vi "Parse Path Object Items.vi"(9 "error in (no error)":errorcluster, 11 "Path with leading Object element":string) -> (1 "error out":errorcluster, 2 "<JSON>items names":string[](array[string]), 3 "Rest or Path":string, 4 "Is Array":bool)   [LabVIEW 2019, in "JSONtext.lvlib"]
uses:
  JSONtext.lvlib
  Parsing State.ctl
  Advance past Line Ending.vi
  support/quote and escape json string 2.vi
  JDP Science Common Utilities/JDP Utility.lvlib
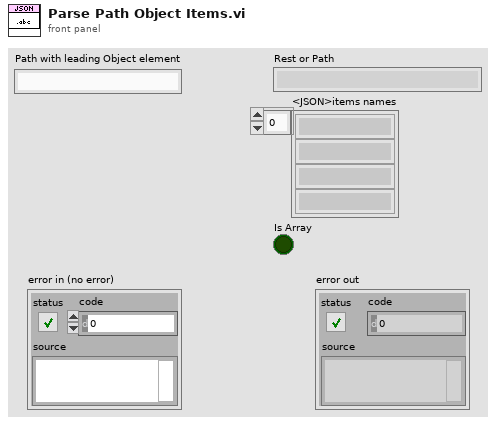
[diagram p1: front panel]
types:
  T1 = typedef "JSONtext.lvlib/Parsing State.ctl" = enum16{"Parser Error", "Object", "Array", "String", "Number/Other", "Leading Whitespace", "Object end", "Array end", "Value end"}
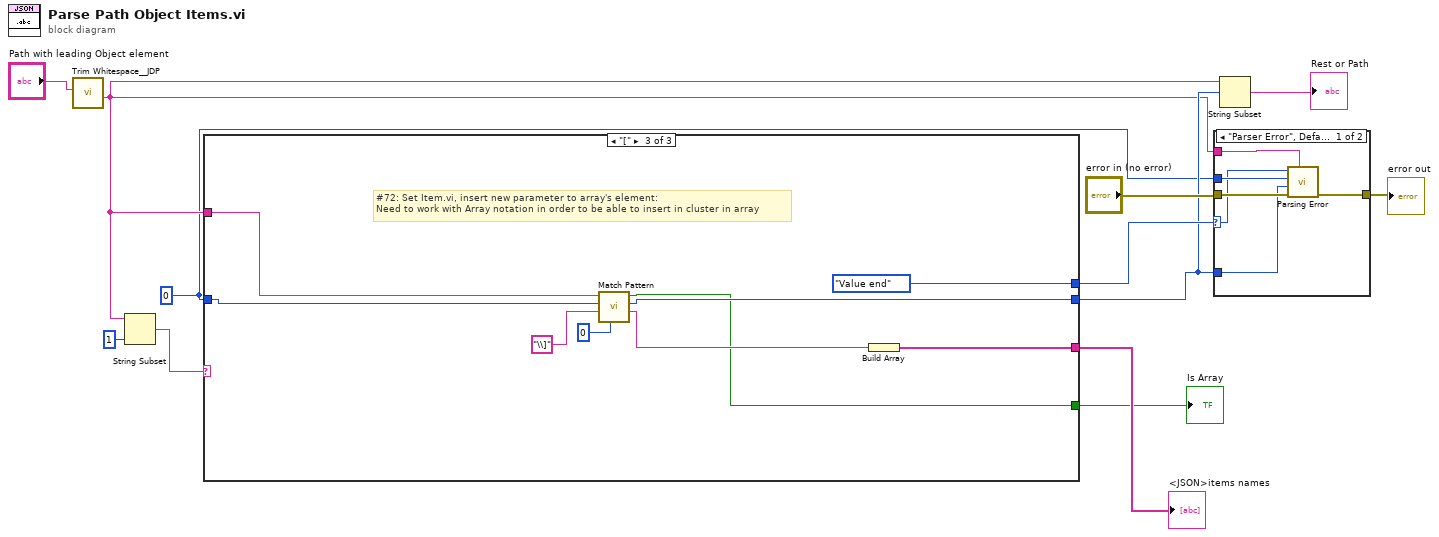
[diagram p0: block diagram]
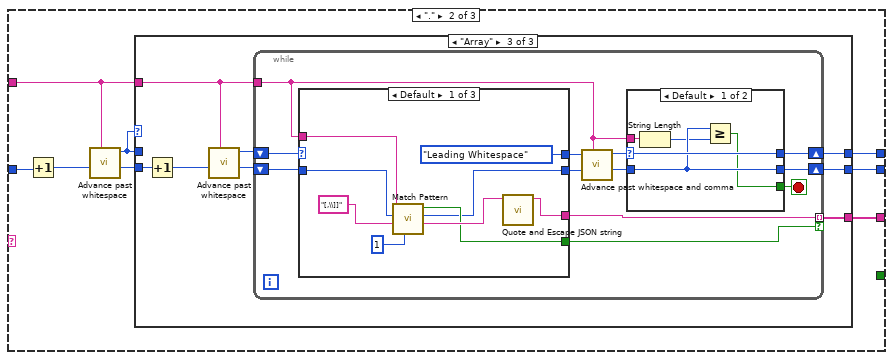
[diagram p4: hidden frame]
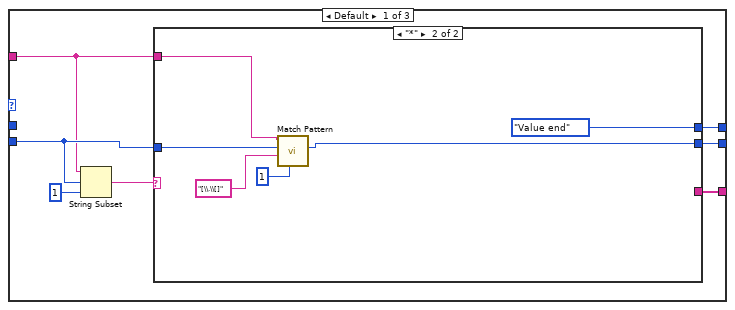
[diagram p5: hidden frame]
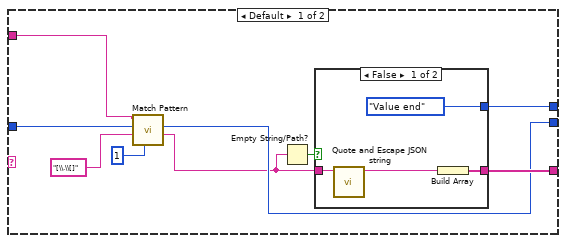
[diagram p6: hidden frame]
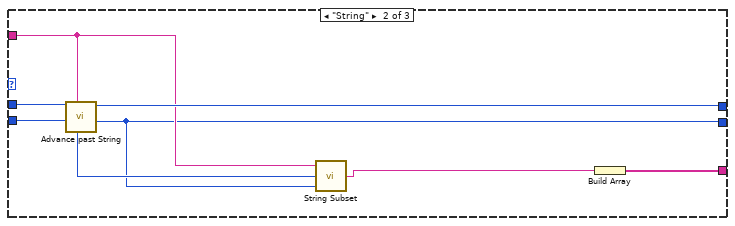
[diagram p8: hidden frame]
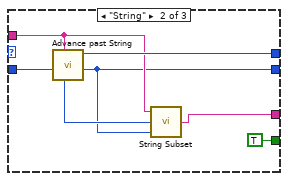
[diagram p9: hidden frame]
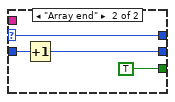
[diagram p11: hidden frame]
diagram:
  w3 = 0
  n1 = call "Trim Whitespace__JDP.vi"("String in"="Path with leading Object element") -> ("String out"=w5:string)  [unwired: 6 in]
  n2 = String Subset(string=w5, length (rest)=1 ("length (rest)")) -> (substring=w2:string)  [unwired: 1 in]
  n3 = case shown="\"[\"" w2 {
    tunnel: w3 -> [w13 w21 w111]
    tunnel: w5 -> [_ w19 w110]
    tunnel: [_ w18 w104] -> w9
    tunnel: [w13 w17 w109] -> w8
    tunnel: [_ w14 Parsing_State."Value end" ("Parser State")] -> w10
    tunnel: [_ _ w103] -> w1
    frame Default {
    }
    frame "." {
      n4 = Increment(x=w21) -> (x+1=w20:i32)
      n5 = call "Advance past whitespace.vi"("JSON"=w19, "Offset"=w20) -> ("Offset of first non-whitespace"=w16:i32, "Parser State"=w15:T1)  [unwired: 7 in, 1 out]
      n6 = case shown="\"Array\"" w15 {
        tunnel: w15 -> [_ w55 _]
        tunnel: w19 -> [w23 w52 w56]
        tunnel: w16 -> [w24 w54 w63]
        tunnel: [w28 w48 w62] -> w18
        tunnel: [w27 w50 w61] -> w17
        tunnel: [w26 w53 w60] -> w14
        frame Default {
          n7 = String Subset(string=w23, offset (0)=w24, length (rest)=1 ("length (rest)")) -> (substring=w22:string)
          n8 = case shown="\"*\"" w22 {
            tunnel: [w37 _] -> w28
            tunnel: [w35 w46] -> w27
            tunnel: [w34 Parsing_State."Value end" ("Parser State")] -> w26
            tunnel: w24 -> [w30 w43]
            tunnel: w23 -> [w29 w42]
            frame Default {
              n9 = call "Match Pattern.vi"("trim back if found"=1, "regular expression"="[\\.\\[]", "Offset in"=w30, "String in"=w29) -> ("substring"=w32:string, "Offset of match"=w35:i32)  [unwired: 5 in, 1 out]
              n10 = Empty String/Path?(string/path=w32) -> (empty?=w33:bool)
              n11 = case shown="False" w33 {
                tunnel: [w40 _] -> w37
                tunnel: w32 -> [w39 _]
                tunnel: [Parsing_State."Value end" ("Parser State") _] -> w34
                frame False {
                  n12 = call "Quote and Escape JSON string.vi"("Plain Text"=w39) -> ("<JSON>"=w41:string)  [unwired: 10 in]
                  n13 = Build Array(w41) -> (w40:string[])
                }
                frame True {
                }
              }
            }
            frame "*" {
              n14 = call "Match Pattern.vi"("trim back if found"=1, "regular expression"="[\\.\\[]", "Offset in"=w43, "String in"=w42) -> ("Offset of match"=w46:i32)  [unwired: 5 in, 2 out]
            }
          }
        }
        frame "String" {
          n15 = call "Advance past String.vi"("JSON"=w52, "Offset"=w54, "State in"=w55) -> ("Offset past match"=w50:i32, "State"=w53:T1, "Value start out"=w51:i32)  [unwired: 6 in]
          n16 = call "String Subset.vi"("Offset past End"=w50, "Start offset"=w51, "JSON"=w52) -> ("substring"=w49:string)  [unwired: 2 in]
          n17 = Build Array(w49) -> (w48:string[])
        }
        frame "Array" {
          n18 = Increment(x=w63) -> (x+1=w57:i32)
          n19 = call "Advance past whitespace.vi"("JSON"=w56, "Offset"=w57) -> ("Offset of first non-whitespace"=w58:i32, "Parser State"=w59:T1)  [unwired: 7 in, 1 out]
          n20 = while {
            tunnel: w56 -> [w65]
            shift-right: [w73] -> w61
            shift-left: w58 -> [w67]
            shift-right: [w69] -> w60
            shift-left: w59 -> [w68]
            tunnel: [w66] -> w62 mode=indexing if=w64
            stop <- w72 stop-if-true
            n21 = case shown="Default" w68 {
              selector: w68 -> [_ _ w93]
              tunnel: w67 -> [w81 w90 w92]
              tunnel: [Parsing_State."Leading Whitespace" ("State") w91 w93] -> w71
              tunnel: [w76 w87 w92] -> w70
              tunnel: w65 -> [w83 w89 _]
              tunnel: [w82 w86 _] -> w66
              tunnel: [w79 TRUE ("Found") _] -> w64
              frame Default {
                n22 = call "Match Pattern.vi"("trim back if found"=1, "regular expression"="[,\\]]", "Offset in"=w81, "String in"=w83) -> ("substring"=w80:string, "Offset of match"=w76:i32, "Found"=w79:bool)  [unwired: 5 in]
                n23 = call "Quote and Escape JSON string.vi"("Plain Text"=w80) -> ("<JSON>"=w82:string)  [unwired: 10 in]
              }
              frame "String" {
                n24 = call "Advance past String.vi"("JSON"=w89, "Offset"=w90) -> ("Offset past match"=w87:i32, "State"=w91:T1, "Value start out"=w88:i32)  [unwired: 7 in]
                n25 = call "String Subset.vi"("Offset past End"=w87, "Start offset"=w88, "JSON"=w89) -> ("substring"=w86:string)  [unwired: 2 in]
              }
              frame "Array end" {
              }
            }
            n26 = call "Advance past whitespace and comma.vi"("JSON"=w65, "Offset"=w70, "State in"=w71) -> ("Offset past match"=w75:i32, "State"=w74:T1)  [unwired: 6 in, 1 out]
            n27 = case shown="Default" w74 {
              selector: w74 -> [w98 w99]
              tunnel: [w94 TRUE] -> w72
              tunnel: w75 -> [w97 w101]
              tunnel: [w97 w100] -> w73
              tunnel: [w98 w99] -> w69
              tunnel: w65 -> [w95 _]
              frame Default {
                n28 = String Length(string=w95) -> (length=w96:i32)
                n29 = Greater Or Equal?(x=w97, y=w96) -> (x >= y?=w94:bool)
              }
              frame "Array end" {
                n30 = Increment(x=w101) -> (x+1=w100:i32)
              }
            }
          }
        }
      }
    }
    frame "[" {
      # "#72: Set Item.vi, insert new parameter to array's element:\nNeed to work with Array notation in order to be able to insert in cluster in array"
      n31 = call "Match Pattern.vi"("trim back if found"=0, "regular expression"="\\]", "Offset in"=w111, "String in"=w110) -> ("substring"=w105:string, "Offset of match"=w109:i32, "Found"=w103:bool)  [unwired: 5 in]
      n32 = Build Array(w105) -> (w104:string[])
    }
  }
  "<JSON>items names" <- w9
  "Is Array" <- w1
  n33 = case shown="\"Parser Error\", Default" w10 {
    selector: w10 -> [w112 _]
    tunnel: w5 -> [w117 _]
    tunnel: "error in (no error)" -> [w116 w118]
    tunnel: [w115 w118] -> w11
    tunnel: w3 -> [w114 _]
    tunnel: w8 -> [w113 _]
    frame "Parser Error", Default {
      n34 = call "Parsing Error.vi"("JSON"=w117, "error in (no error)"=w116, "Offset past match"=w113, "Value start"=w114, "State"=w112) -> ("error out"=w115:errorcluster)  [unwired: 6 in]
    }
    frame "Array end", "Value end" {
    }
  }
  "error out" <- w11
  n35 = String Subset(string=w5, offset (0)=w8) -> (substring=→"Rest or Path":string)  [unwired: 1 in]
